vi "final.vi"() -> ()   [LabVIEW 2018]
uses:
  <vilib>/Instr/_visa.llb/VISA Configure Serial Port (Instr).vi
panel:
  out "写缓冲区":string
  out "Z":string
  in  "Z":bool
  in  "Y":bool
  in  "X":bool
  in  "文件路径":path=path "C:/Users/Twsa/Documents/Graduction-Project/3Dprinter_labview/gcode_exe/fileFinal.txt"
  in  "端口":refnum<visa-resource-name>="COM4"
  in  "停止":bool
  out "读缓冲区":string
  out "Speed":string
  out "Y":string
  out "X":string
  in  "启用终止符":bool
  in  "flow control":u16(ring) caption="流程控制" items=["无"=0, "XON/XOFF"=1, "RTS/CTS"=2, "DTR/DSR"=4]
  in  "stop bits":u16(ring)=10 caption="停止位" items=["1.0"=10, "1.5"=15, "2.0"=20]
  in  "parity":u16(ring) caption="奇偶" items=["无", "奇", "偶", "标记", "空格"]
  in  "data bits":u16=8 caption="数据比特" min=5 max=8 step=1
  in  "baud rate":u32=9600 caption="波特率"
  # "串口设置"
  # "实时数据操作"
  # "发送设置"
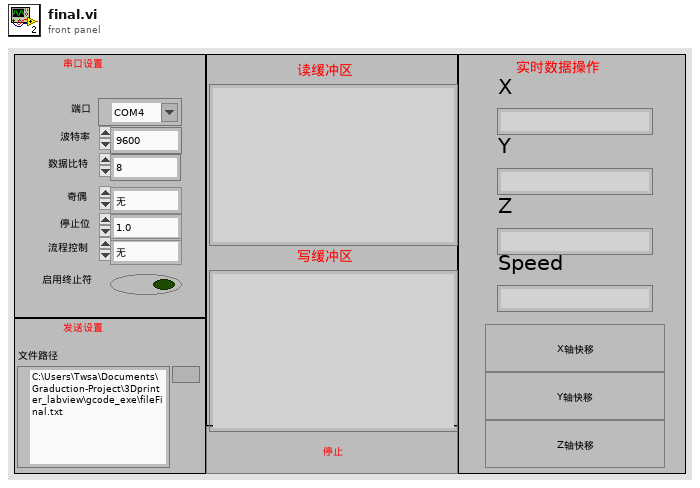
[diagram p1: front panel]
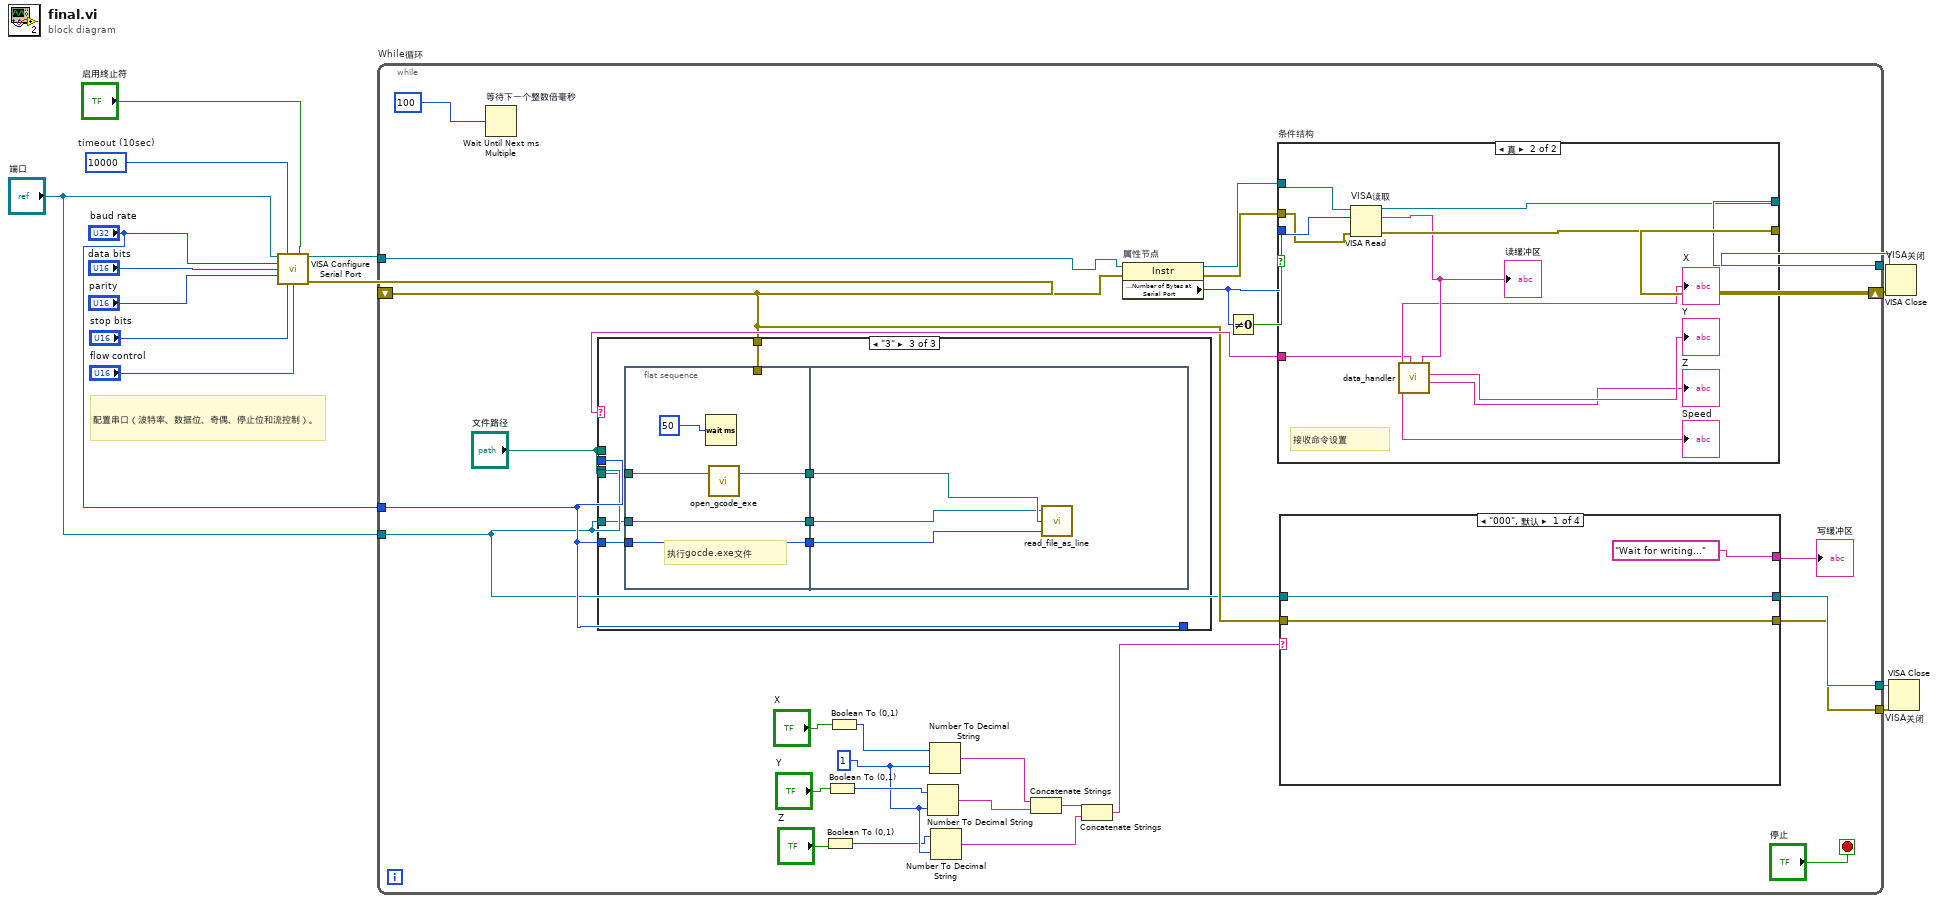
[diagram p0: block diagram]
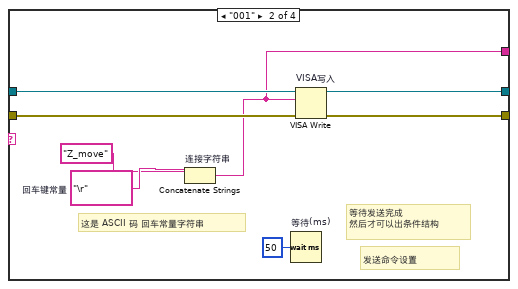
[diagram p2: hidden frame]
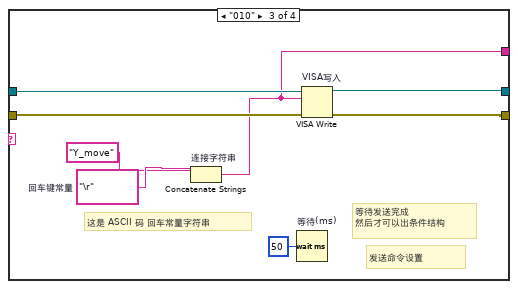
[diagram p3: hidden frame]
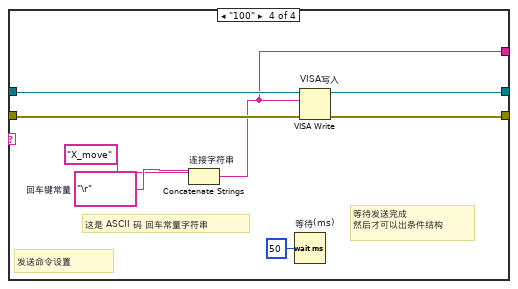
[diagram p4: hidden frame]
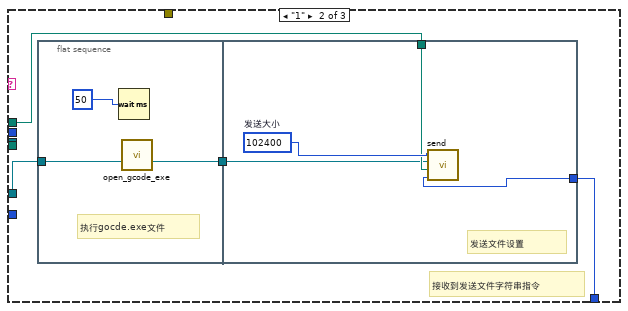
[diagram p6: hidden frame]
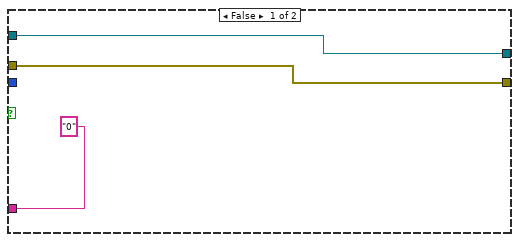
[diagram p7: hidden frame]
diagram:
  w13 = u32 10000  # timeout (10sec)
  # "配置串口（波特率、数据位、奇偶、停止位和流控制）。"
  n1 = call-poly "VISA Configure Serial Port"("VISA resource name"="端口", "timeout (10sec)"=w13, "Enable Termination\nChar (T)"="启用终止符", "baud rate (9600)"="baud rate", "data bits (8)"="data bits", "parity (0:none)"="parity", "stop bits (10: 1 bit)"="stop bits", "flow control (0:none)"="flow control") -> ("VISA resource name out"=w6:refnum<visa-resource-name>, "error out"=w5:errorcluster)  [unwired: 1 in, 5 out]
  n2 = while "While循环" {
    shift-right: [w38] -> w8
    shift-left: w5 -> [w18]
    tunnel: [w35] -> w7
    tunnel: w6 -> [w36]
    tunnel: "端口" -> [w15]
    tunnel: "baud rate" -> [w16]
    tunnel: [w17] -> w2
    tunnel: [w34] -> w1
    stop <- "停止" stop-if-true
    w28 = 1
    n3 = Wait Until Next ms Multiple "等待下一个整数倍毫秒"(millisecond multiple=u32 100 ("毫秒倍数")) -> ()  [unwired: 1 out]
    n4 = Boolean To (0,1)(Boolean="Z") -> (0, 1=w27:i16)
    n5 = Boolean To (0,1)(Boolean="Y") -> (0, 1=w29:i16)
    n6 = Boolean To (0,1)(Boolean="X") -> (0, 1=w30:i16)
    n7 = Number To Decimal String(number=w29, width (-)=w28) -> (decimal integer string=w25:string)
    n8 = Number To Decimal String(number=w30, width (-)=w28) -> (decimal integer string=w26:string)
    n9 = Number To Decimal String(number=w27, width (-)=w28) -> (decimal integer string=w23:string)
    n10 = Concatenate Strings(w26, w25) -> (w24:string)
    n11 = Concatenate Strings(w24, w23) -> (w22:string)
    n12 = property on="属性节点" class="Instr"(reference=w36, error in=w18) -> (reference out=w39:refnum<visa-resource-name>, error out=w37:errorcluster, "Serial Settings:Number of Bytes at Serial Port"=w40:u32)
    n13 = Not Equal To 0?(x=w40) -> (x != 0?=w41:bool)
    n14 = case "条件结构" shown="真" w41 {
      tunnel: w40 -> [_ w108]
      tunnel: w39 -> [w97 w107]
      tunnel: [w96 w106] -> w38
      tunnel: [w97 w105] -> w35
      tunnel: w37 -> [w96 w104]
      tunnel: ["0" w98] -> w20
      frame False {
      }
      frame True {
        # "接收命令设置"
        n15 = VISA Read "VISA读取"(VISA resource name=w107, byte count=w108, error in (no error)=w104) -> (VISA resource name out=w105:refnum<visa-resource-name>, read buffer=w103:string, error out=w106:errorcluster)  [unwired: 1 out]
        "读缓冲区" <- w103
        n16 = call "data_handler.vi"("字符串"=w103) -> ("X"=→"X":string, "Y"=→"Y":string, "Z"=→"Z":string, "Speed"=→"Speed":string, "Command"=w98:string)
      }
    }
    n17 = case shown="\"3\"" w20 {
      tunnel: w15 -> [_ _ _]
      tunnel: w16 -> [_ _ _]
      tunnel: w16 -> [_ w74 _]
      tunnel: "文件路径" -> [_ w73 _]
      tunnel: "文件路径" -> [_ _ w87]
      tunnel: w18 -> [_ _ w85]
      tunnel: w16 -> [_ _ w84]
      tunnel: w15 -> [_ w72 w82]
      frame "0", Default {
      }
      frame "1" {
        # "接收到发送文件字符串指令"
        n18 = flat-sequence {
          tunnel: w72 -> [w75]
          tunnel: [w75] -> w71
          tunnel: w74 -> [w79]
          tunnel: w73 -> [w78]
          tunnel: w71 -> [w77]
          frame #0 {
            # "执行gocde.exe文件"
            n19 = Wait (ms)(milliseconds to wait=50) -> ()  [unwired: 1 out]
            n20 = call "open_gcode_exe.vi"() -> ()  [unwired: 1 in]
          }
          frame #1 {
            w80 = 102400  # 发送大小
            # "发送文件设置"
            n21 = call "send.vi"("baud rate"=w79, "文件路径"=w78, "端口"=w77, "数值"=w80) -> ()
          }
        }
      }
      frame "3" {
        n22 = flat-sequence {
          tunnel: w87 -> [w90]
          tunnel: [w90] -> w86
          tunnel: w85 -> [_]
          tunnel: w84 -> [w89]
          tunnel: [w89] -> w83
          tunnel: w82 -> [w88]
          tunnel: [w88] -> w81
          tunnel: w86 -> [w94]
          tunnel: w83 -> [w93]
          tunnel: w81 -> [w92]
          frame #0 {
            # "执行gocde.exe文件"
            n23 = Wait (ms)(milliseconds to wait=50) -> ()  [unwired: 1 out]
            n24 = call "open_gcode_exe.vi"() -> ()  [unwired: 1 in]
          }
          frame #1 {
            n25 = call "read_file_as_line.vi"("baud rate"=w93, "路径"=w94, "端口"=w92) -> ()
          }
        }
      }
    }
    n26 = case shown="\"000\", 默认" w22 {
      tunnel: w15 -> [w46 w52 w57 w66]
      tunnel: w18 -> [w45 w51 w58 w67]
      tunnel: [w45 w50 w60 w64] -> w17
      tunnel: [w46 w49 w59 w65] -> w34
      tunnel: ["Wait for writing..." w47 w55 w63] -> w21
      frame "000", Default {
      }
      frame "001" {
        w53 = "\r"  # 回车键常量
        # "发送命令设置"
        # "等待发送完成\n然后才可以出条件结构"
        # "这是 ASCII 码 回车常量字符串"
        n27 = Concatenate Strings "连接字符串"("Z_move", w53) -> (w47:string)
        n28 = Wait (ms) "等待(ms)"(milliseconds to wait=u32 50) -> ()  [unwired: 1 out]
        n29 = VISA Write "VISA写入"(VISA resource name=w52, write buffer=w47, error in (no error)=w51) -> (VISA resource name out=w49:refnum<visa-resource-name>, error out=w50:errorcluster)  [unwired: 1 out]
      }
      frame "010" {
        w61 = "\r"  # 回车键常量
        # "发送命令设置"
        # "等待发送完成\n然后才可以出条件结构"
        # "这是 ASCII 码 回车常量字符串"
        n30 = Concatenate Strings "连接字符串"("Y_move", w61) -> (w55:string)
        n31 = Wait (ms) "等待(ms)"(milliseconds to wait=u32 50) -> ()  [unwired: 1 out]
        n32 = VISA Write "VISA写入"(VISA resource name=w57, write buffer=w55, error in (no error)=w58) -> (VISA resource name out=w59:refnum<visa-resource-name>, error out=w60:errorcluster)  [unwired: 1 out]
      }
      frame "100" {
        w69 = "\r"  # 回车键常量
        # "发送命令设置"
        # "等待发送完成\n然后才可以出条件结构"
        # "这是 ASCII 码 回车常量字符串"
        n33 = Concatenate Strings "连接字符串"("X_move", w69) -> (w63:string)
        n34 = Wait (ms) "等待(ms)"(milliseconds to wait=u32 50) -> ()  [unwired: 1 out]
        n35 = VISA Write "VISA写入"(VISA resource name=w66, write buffer=w63, error in (no error)=w67) -> (VISA resource name out=w65:refnum<visa-resource-name>, error out=w64:errorcluster)  [unwired: 1 out]
      }
    }
    "写缓冲区" <- w21
  }
  n36 = VISA Close "VISA关闭"(VISA resource name=w7, error in (no error)=w8) -> ()  [unwired: 1 out]
  n37 = VISA Close "VISA关闭"(VISA resource name=w1, error in (no error)=w2) -> ()  [unwired: 1 out]
